vi "Configuration 2.0 JSON Flatten.vi"(8 "error in (no error)":errorcluster, 11 "dsf configuration 2.0":T2) -> (0 "error out":errorcluster, 2 "dsf version":T1, 3 "dsf configuration json":string)   [LabVIEW 2017, in "DSF Core.lvlib" / "Configuration Session.lvclass"]
uses:
  Configuration Session.lvclass
  Typedefs/DSF Version Info.ctl
  DSF Core.lvlib
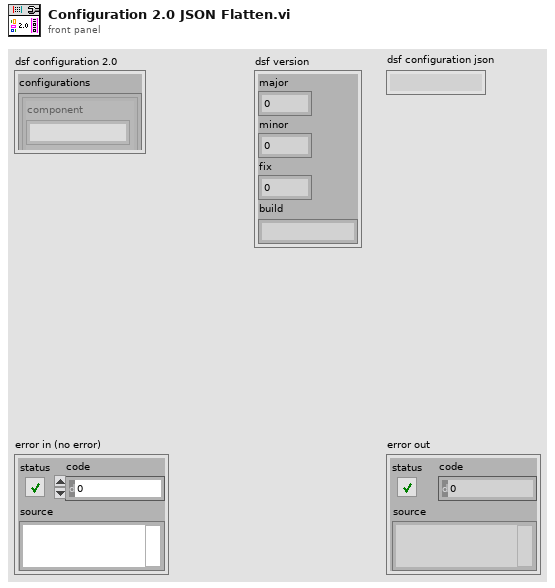
[diagram p1: front panel]
types:
  T1 = typedef "DSF Core.lvlib/DSF Version Info.ctl" = cluster{"major":i32, "minor":i32, "fix":i32, "build":string}
  T2 = cluster{"configurations":cluster{"component":string, "data":string, "data version":cluster{"major":i32, "minor":i32, "fix":i32, "build":string}}[], "plugins":cluster{"configurations":cluster{"component":string, "data":string, "data version":cluster{"major":i32, "minor":i32, "fix":i32, "build":string}}[], "threads":cluster{"configurations":cluster{"component":string, "data":string, "data version":cluster{"major":i32, "minor":i32, "fix":i32, "build":string}}[], "groups":cluster{"configurations":cluster{"component":string, "data":string, "data version":cluster{"major":i32, "minor":i32, "fix":i32, "build":string}}[], "transfers":cluster{"configurations":cluster{"component":string, "data":string, "data version":cluster{"major":i32, "minor":i32, "fix":i32, "build":string}}[]}[]}[]}[]}[]}
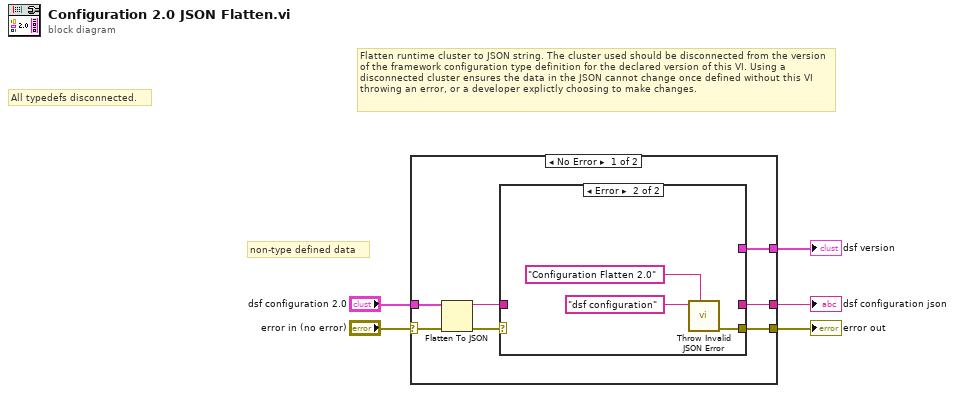
[diagram p0: block diagram]
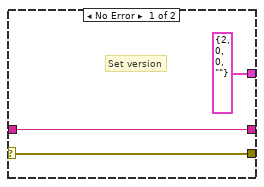
[diagram p2: hidden frame]
diagram:
  # "non-type defined data"
  # "All typedefs disconnected."
  # "Flatten runtime cluster to JSON string. The cluster used should be disconnected from the version of the framework configuration type definition for the declared version of this VI. Using a disconnected cluster ensures the data in the JSON cannot change once defined without this VI throwing an error, or a developer explictly choosing to make changes."
  n1 = case shown="No Error" "error in (no error)" {
    selector: "error in (no error)" -> [w9 w19]
    tunnel: [w11 w19] -> w5
    tunnel: "dsf configuration 2.0" -> [w8 _]
    tunnel: [w7 _] -> w2
    tunnel: [w6 _] -> w1
    frame No Error {
      n2 = Flatten To JSON(anything=w8, error in (no error)=w9) -> (JSON string=w10:string, 11:w12:errorcluster)  [unwired: 1 in]
      n3 = case shown="Error" w12 {
        selector: w12 -> [w15 _]
        tunnel: [w15 w18] -> w11
        tunnel: w10 -> [w14 _]
        tunnel: [w14 _] -> w7
        tunnel: [T1 {"major"=2, "minor"=0, "fix"=0, "build"=""} ("json version") _] -> w6
        frame No Error {
          # "Set version"
        }
        frame Error {
          n4 = call "Throw Invalid JSON Error.vi"("error source vi name"="Configuration Flatten 2.0", "name"="dsf configuration") -> ("error out"=w18:errorcluster)  [unwired: 9 in]
        }
      }
    }
    frame Error {
    }
  }
  "dsf configuration json" <- w2
  "error out" <- w5
  "dsf version" <- w1
